vi "TSI Bench Single Socket CPV Sweeps Ver1.0.vi"() -> ()   [LabVIEW 2017]
uses:
  <vilib>/Utility/file.llb/Read Delimited Spreadsheet (DBL).vi
  <instrlib>/Agilent E364X Series/Agilent E364X Series.lvlib
  <instrlib>/Agilent E4980/Agilent E4980.lvlib
  <instrlib>/Keithley 2000/Keithley 2000.lvlib
panel:
  out "Cycles":string="2000"
  in  "Tab Control":enum32{"Control"}(tab)
  in  "T- CAP(fF)":dbl[](array[numeric])=[100.0, 2968.75]
  out "Diff DCAP":dbl[](array[numeric])=[0.0, 158.76451612903202, 128.65967741935475, 83.51039999999999, 79.098, 80.17639999999999, 81.14560000000002, 79.77199999999999, 91.06439999999998, 80.7144, 80.3784, 79.76879999999998, 80.59799999999998, 91.3732, 90.2772]
  out "IDD ON (uA)":string
  out "I_Stdby (uA)":string
  out "CMax(fF)":dbl
  in  "Cycle?":bool=TRUE
  out "Cycles  No":i32=2000
  out "CMin (fF)":dbl=255.30700000000002
  in  "TP":string="TSI Bench Single Socket CPV Sweep Ver1.0"
  out "Error Out":errorcluster={"status"=FALSE, "code"=1073676407, "source"="VISA Open in Agilent E364X Series.lvlib:Initialize.vi->WS1021 Screen Parts Bench Test Ver1.4.vi"}
  in  "Base Path":path=path "C:/TSI Material"
  out "Status":string="Save Data..."
  in  "Tab Control 2":T1(tab)=enum."Input Info"
  in  "AGE364X":refnum<visa-resource-name>="GPIB0::6::INSTR"
  in  "VDD/VIO":dbl[](array[numeric])=[3.3, 1.8]
  in  "I_Limit (mA)":dbl=20.0 format="%.2p"
  in  "Select CPV":i32(ring)=17 items=["CP 24V", "CP 26V", "CP 28V", "CP 30V", "CP 31V", "CP 32V", "CP 33V", "CP 34V", "CP 35V", "CP 36V", "CP 37V", "CP 38V", "CP 39V", "CP 40V", "CP 41V", "CP 42V", "CP 43V", "CP 44V", "CP 45V", "CP 46V", "CP 47V", "CP 48V", "CP 49V", "CP 50V", "CP 51V", "CP 52V", "CP 53V", "CP 54V", "CP 56V", "CP 58V", "CP 60V", "CP 62V"]
  in  "Settings":bool
  in  "Comport Setting":refnum<visa-resource-name>="COM8"
  in  "Manual Write":string
  in  "Send":bool
  in  "No of Cycles":i32=2000
  in  "Type (0: Cp-D)":u16(ring)=1 items=["Cp-D", "Cp-Q", "Cp-G", "Cp-Rp", "Cs-D", "Cs-Q", "Cs-Rs", "Lp-D", "Lp-Q", "Lp-G", "Lp-Rp", "Ls-D", "Ls-Q", "Ls-Rs", "R-X", "Z-thd", "Z-thr", "G-B", "Y-thd", "Y-thr"]
  in  "Auto Range":bool=TRUE
  in  "AG4980A":refnum<visa-resource-name>="GPIB0::17::INSTR"
  in  "KE2000":refnum<visa-resource-name>="GPIB0::9::INSTR"
  in  "Process Stop Button":bool
  in  "Read X, Y Setting":string[](array[string])=["68", "69"]
  in  "Stop":bool
  in  "Error In":errorcluster
  in  "CP CYC":bool
  in  "VDD":bool
  in  "Capacitance":bool
  in  "Info":T2={"Lot"="3127C", "Wafer"="11", "Package"="BC_C", "Device"="1"}
  out "IDD":cluster{dbl[], dbl[]}(graph)
  out "Cap Plot":cluster{dbl[], dbl[]}(graph)
  # "WiSpry Inc 20 Fairbanks \nSte 198 Irvine CA 92618\n\n\n\n\nRev Date = 11/11/2020\nTP:  TSI Bench Single Socket CPV Sweep Ver1.0\nLabVIEW 2017"
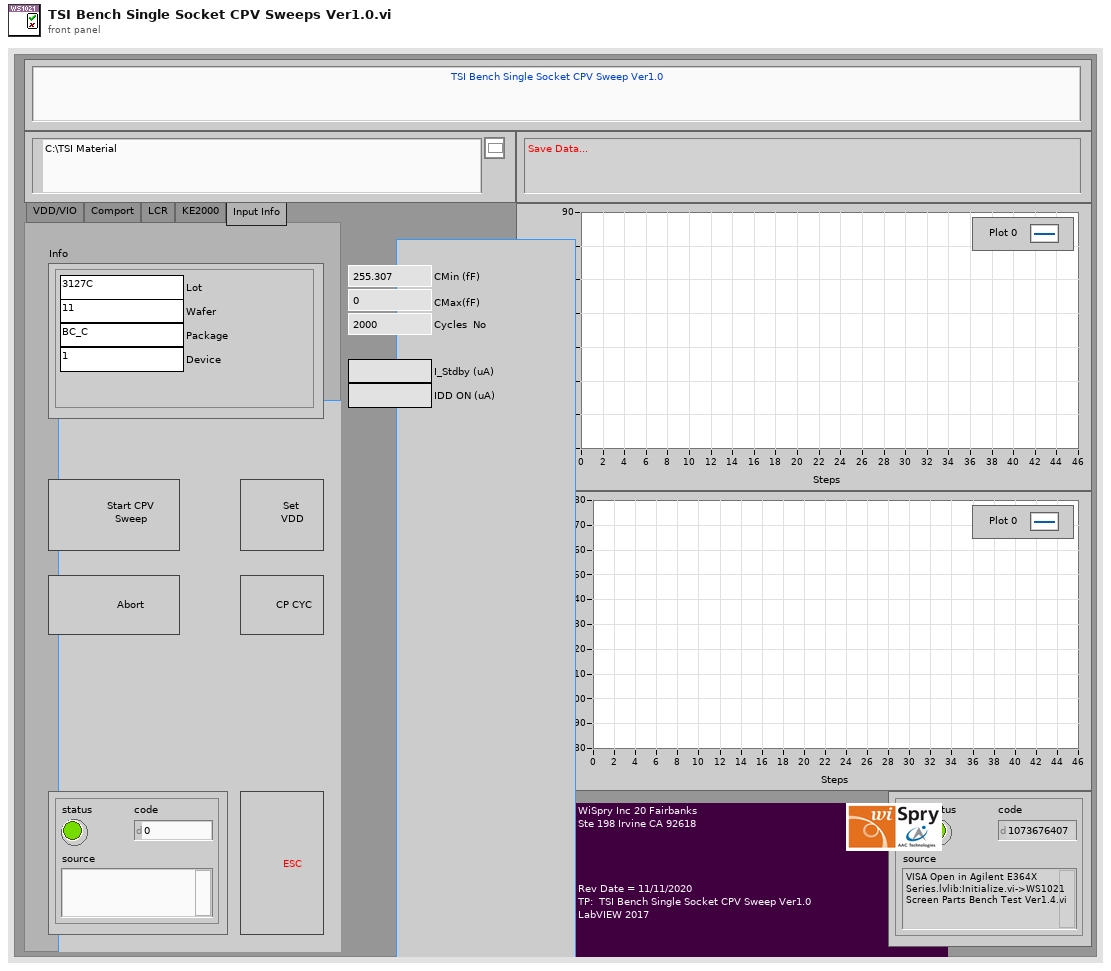
[diagram p1: front panel]
types:
  T1 = enum32{"VDD/VIO", "Comport", "LCR", "KE2000", "Input Info"}
  T2 = cluster{"Lot":string, "Wafer":string, "Package":string, "Device":string}
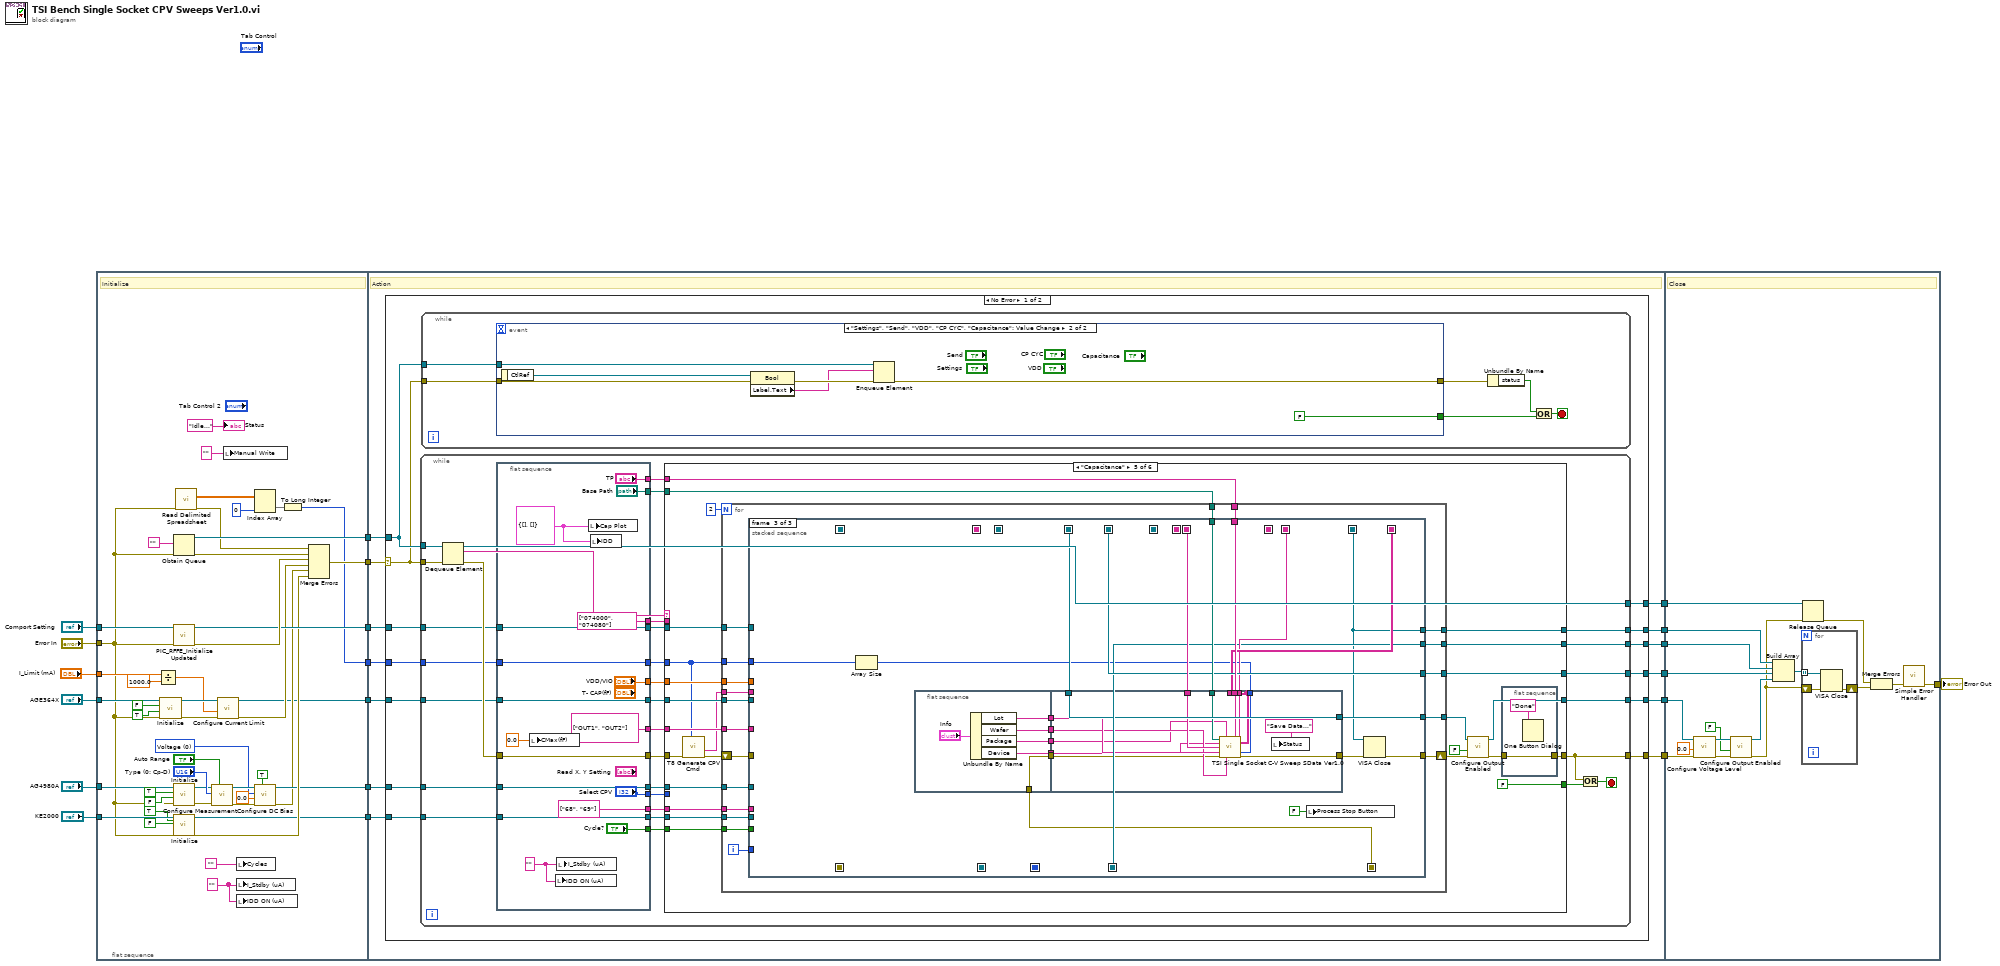
[diagram p0: block diagram]
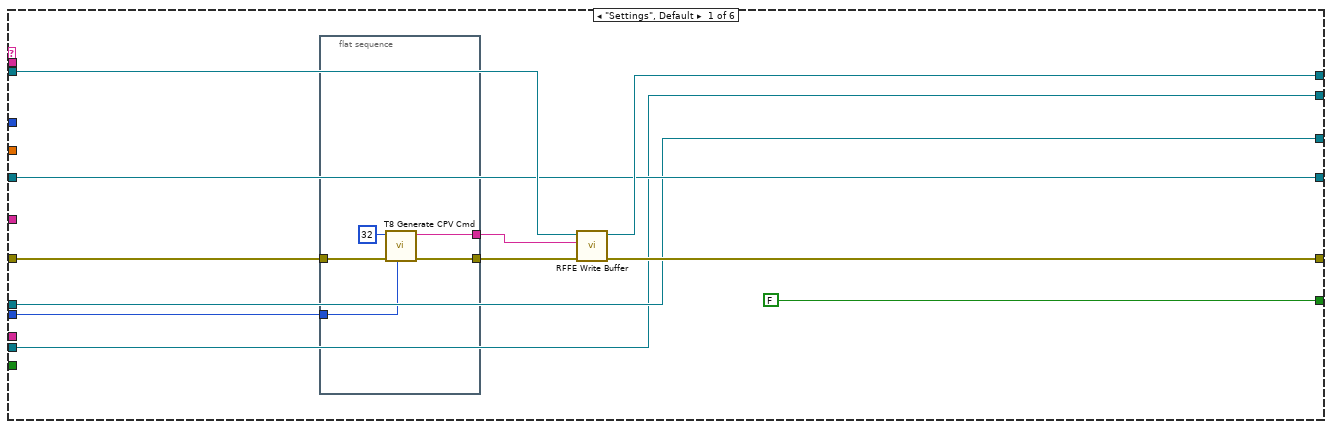
[diagram p2: hidden frame]
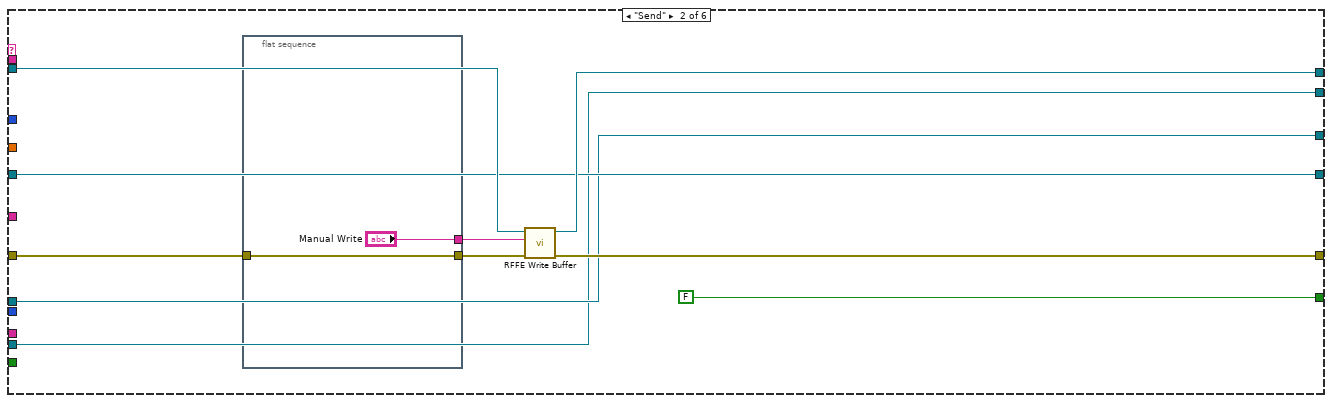
[diagram p3: hidden frame]
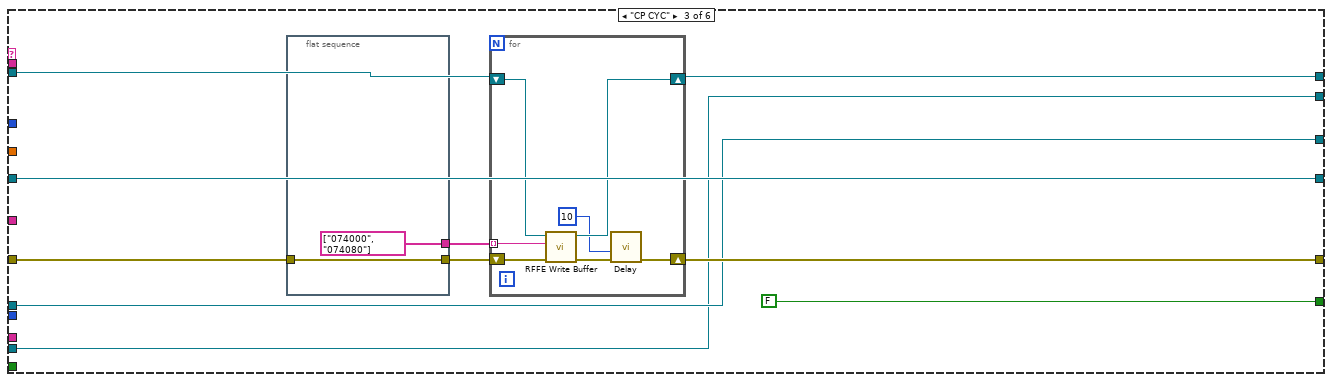
[diagram p4: hidden frame]
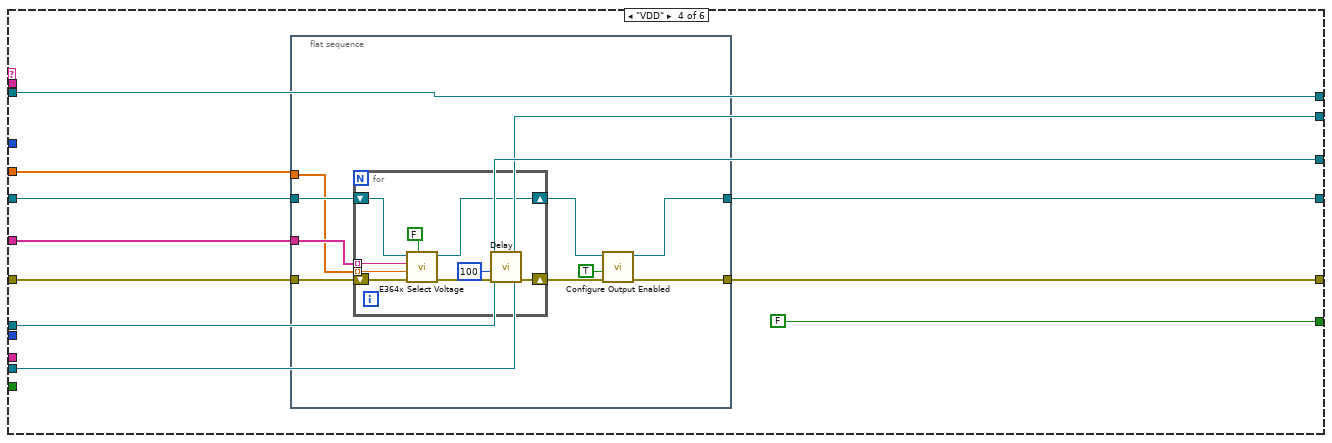
[diagram p5: hidden frame]
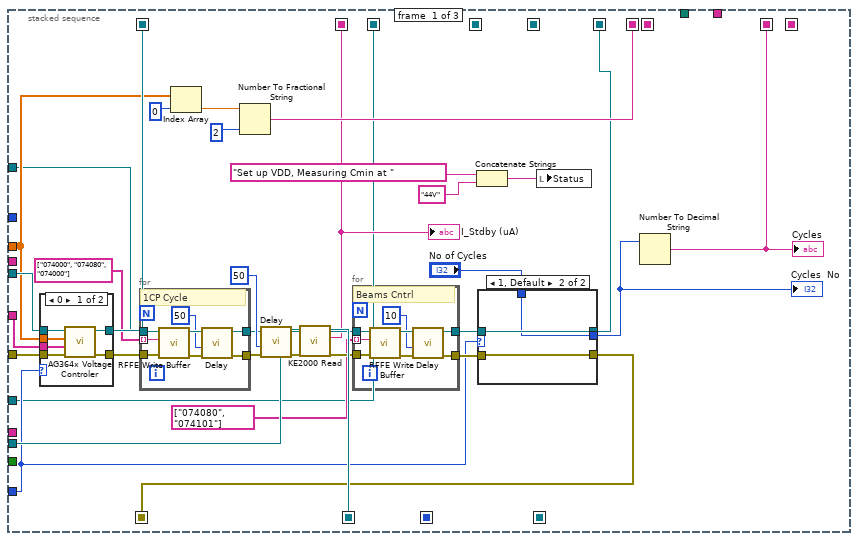
[diagram p6: hidden frame]
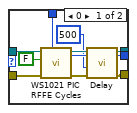
[diagram p8: hidden frame]
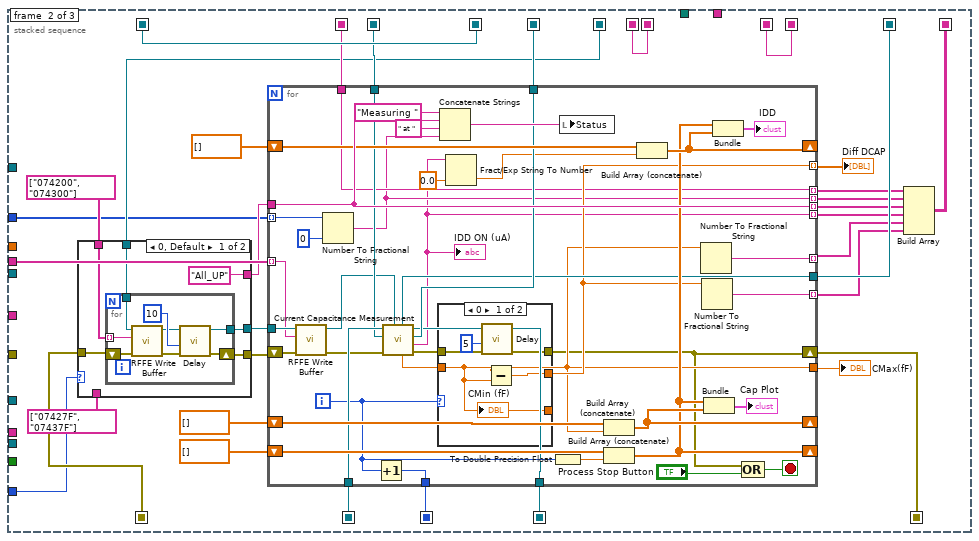
[diagram p9: hidden frame]
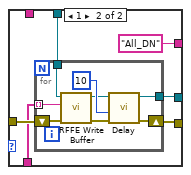
[diagram p10: hidden frame]
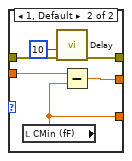
[diagram p11: hidden frame]
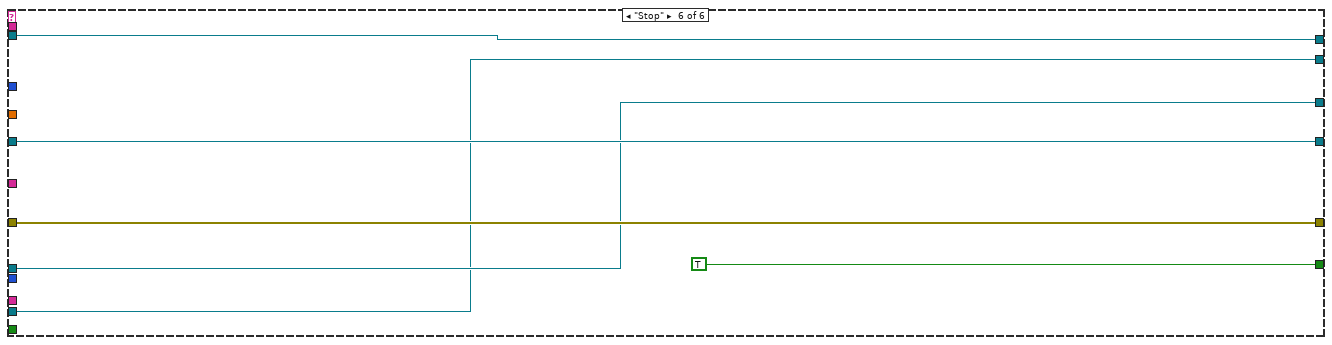
[diagram p12: hidden frame]
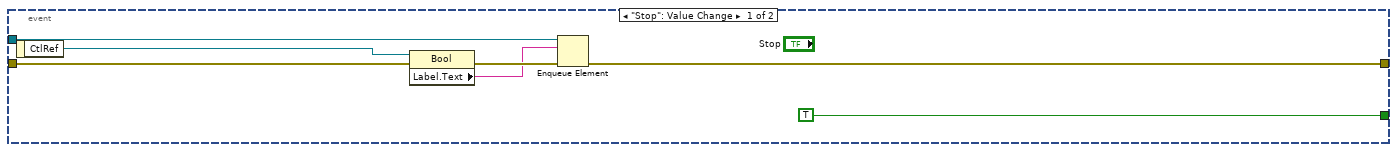
[diagram p13: hidden frame]
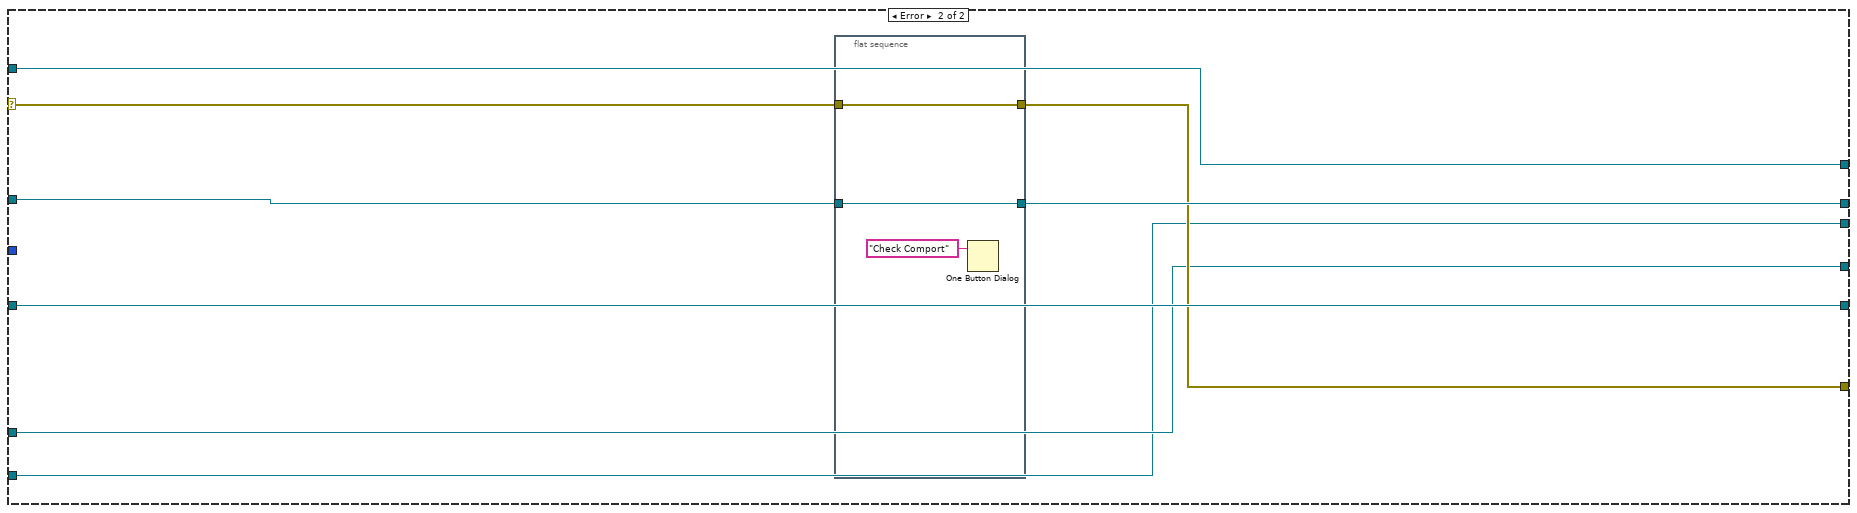
[diagram p14: hidden frame]
diagram:
  n1 = flat-sequence {
    tunnel: "Error In" -> [w23]
    tunnel: [w63] -> w19
    tunnel: [w65] -> w18
    tunnel: "Comport Setting" -> [w64]
    tunnel: [w60] -> w15
    tunnel: "AGE364X" -> [w58]
    tunnel: [w31] -> w11
    tunnel: "AG4980A" -> [w49]
    tunnel: [w41] -> w7
    tunnel: "KE2000" -> [w45]
    tunnel: [w42] -> w4
    tunnel: "I_Limit (mA)" -> [w30]
    tunnel: [w21] -> w1
    tunnel: w19 -> [w75]
    tunnel: w18 -> [w79]
    tunnel: [w78] -> w17
    tunnel: w15 -> [w77]
    tunnel: [w76] -> w14
    tunnel: w11 -> [w74]
    tunnel: [w73] -> w10
    tunnel: [w72] -> w9
    tunnel: w7 -> [w71]
    tunnel: [w70] -> w6
    tunnel: w4 -> [w69]
    tunnel: [w68] -> w3
    tunnel: w1 -> [w67]
    tunnel: w17 -> [w533]
    tunnel: w14 -> [w519]
    tunnel: [w532] -> w13
    tunnel: w10 -> [w528]
    tunnel: w9 -> [w524]
    tunnel: w6 -> [w521]
    tunnel: w3 -> [w518]
    frame #0 {
      w27 = "" ("I_Stdby (uA)")
      w38 = u16 0 items=["Voltage", "Current"] ("DC Bias Type (0: Voltage)")
      # "Initialize"
      n2 = Divide(x=w30, y=1000.0) -> (x/y=w28:dbl)
      n3 = call <instrlib>:"Initialize.vi"("error in (no error)"=w23, "ID Query (T: Query)"=TRUE, "Reset Device (T: Reset)"=FALSE, "VISA resource name"=w58) -> ("error out"=w33:errorcluster, "VISA resource name out"=w34:refnum<visa-resource-name>)  [unwired: 6 in]
      n4 = Obtain Queue(element data type="", error in (no error)=w23) -> (queue out=w65:refnum<queue>, error out=w62:errorcluster)  [unwired: 3 in, 1 out]
      n5 = call "PIC_RFFE_Initialize Updated.vi"("error in"=w23, "VISA In"=w64) -> ("error out"=w61:errorcluster, "VISA Out"=w60:refnum<visa-resource-name>)  [unwired: 8 in]
      n6 = call <instrlib>:"Initialize.vi"("error in (no error)"=w23, "Reset (True)"=FALSE, "ID Query (True)"=TRUE, "VISA resource name"=w49) -> ("error out"=w53:errorcluster, "VISA resource name out"=w52:refnum<visa-resource-name>)  [unwired: 6 in]
      n7 = call <instrlib>:"Initialize.vi"("VISA resource name"=w45, "ID Query? (T: Check)"=TRUE, "Reset? (T: Reset)"=FALSE, "error in (no error)"=w23) -> ("VISA resource name out"=w42:refnum<visa-resource-name>, "error out"=w46:errorcluster)  [unwired: 14 in]
      n8 = call-poly <vilib>:"Read Delimited Spreadsheet.vi"("error in (no error)"=w23) -> ("all rows"=w26:dbl[][], "error out"=w22:errorcluster)  [unwired: 9 in, 4 out]
      n9 = call <instrlib>:"Configure Measurement.vi"("Enable Auto Range (T:Enable)"="Auto Range", "error in (no error)"=w53, "Function (0: Cp-D)"="Type (0: Cp-D)", "VISA resource name"=w52) -> ("error out"=w37:errorcluster, "VISA resource name out"=w40:refnum<visa-resource-name>)  [unwired: 6 in]
      n10 = call <instrlib>:"Configure Current Limit.vi"("error in (no error)"=w33, "Current Limit (0.0 Amps)"=w28, "VISA resource name"=w34) -> ("error out"=w32:errorcluster, "VISA resource name out"=w31:refnum<visa-resource-name>)  [unwired: 7 in]
      n11 = local write "Manual Write"("" ("Manual Write")) -> ()
      n12 = local write "Cycles"("") -> ()
      n13 = local write "I_Stdby (uA)"(w27) -> ()
      n14 = local write "IDD ON (uA)"(w27) -> ()
      n15 = Index Array(array=w26, index (col)=0 ("disabled index (col)")) -> (element=w24:dbl[])  [unwired: 1 in]
      n16 = call <instrlib>:"Configure DC Bias.vi"("DC Bias State (F:Disable)"=TRUE, "error in (no error)"=w37, "DC Bias Level (0.0 V)"=0.0, "DC Bias Type (0: Voltage)"=w38, "VISA resource name"=w40) -> ("error out"=w36:errorcluster, "VISA resource name out"=w41:refnum<visa-resource-name>)  [unwired: 5 in]
      n17 = To Long Integer(number=w24) -> (32bit integer=w21:i32[])
      n18 = Merge Errors(w22, w62, w61, w32, w36, w46) -> (w63:errorcluster)
      "Status" <- "Idle..." ("Status")
    }
    frame #1 {
      # "Action"
      n19 = case shown="No Error" w75 {
        selector: w75 -> [w88 w509]
        tunnel: w79 -> [w92 w511]
        tunnel: [w91 w511] -> w78
        tunnel: w77 -> [w90 w513]
        tunnel: [w89 w512] -> w76
        tunnel: w74 -> [w87 w510]
        tunnel: [w86 w508] -> w73
        tunnel: [w85 w510] -> w72
        tunnel: w71 -> [w84 w507]
        tunnel: [w83 w507] -> w70
        tunnel: w69 -> [w82 w506]
        tunnel: [w81 w506] -> w68
        tunnel: w67 -> [w80 _]
        frame No Error {
          n20 = while {
            tunnel: w92 -> [w123]
            tunnel: w88 -> [w122]
            tunnel: [w116] -> w91
            tunnel: w90 -> [w115]
            tunnel: [w113] -> w89
            tunnel: w87 -> [w112]
            tunnel: [w109] -> w85
            tunnel: [w104] -> w86
            tunnel: w84 -> [w107]
            tunnel: [w105] -> w83
            tunnel: w82 -> [w100]
            tunnel: [w98] -> w81
            tunnel: w80 -> [w94]
            stop <- w118 stop-if-true
            n21 = Dequeue Element(queue=w123, error in (no error)=w122) -> (queue out=w116:refnum<queue>, element=w121:string, error out=w120:errorcluster)  [unwired: 1 in, 1 out]
            n22 = flat-sequence {
              tunnel: w120 -> [w485]
              tunnel: [w485] -> w119
              tunnel: w115 -> [w484]
              tunnel: [w484] -> w114
              tunnel: w112 -> [w483]
              tunnel: [w483] -> w111
              tunnel: [string[] ["OUT1", "OUT2"]] -> w110
              tunnel: ["VDD/VIO"] -> w108
              tunnel: w107 -> [w481]
              tunnel: [w481] -> w106
              tunnel: ["Base Path"] -> w103
              tunnel: ["TP"] -> w102
              tunnel: ["Select CPV"] -> w101
              tunnel: w100 -> [w477]
              tunnel: [w477] -> w99
              tunnel: [string[] ["074000", "074080"]] -> w97
              tunnel: ["Cycle?"] -> w96
              tunnel: [string[] ["68", "69"]] -> w95
              tunnel: [w470] -> w93
              tunnel: w94 -> [w470]
              frame #0 {
                w472 = "" ("I_Stdby (uA)")
                w473 = cluster{dbl[], dbl[]} {[], []} ("Cap Plot")
                n23 = local write "CMax(fF)"(0.0 ("CMax(fF)")) -> ()
                n24 = local write "IDD ON (uA)"(w472) -> ()
                n25 = local write "I_Stdby (uA)"(w472) -> ()
                n26 = local write "Cap Plot"(w473) -> ()
                n27 = local write "IDD"(w473) -> ()
              }
            }
            n28 = case shown="\"Capacitance\"" w121 {
              tunnel: w119 -> [w134 w146 w158 w178 w203 w468]
              tunnel: [w131 w149 w161 w177 w206 w468] -> w104
              tunnel: [FALSE FALSE FALSE FALSE FALSE TRUE] -> w117
              tunnel: w114 -> [w130 w147 w159 w179 w217 w466]
              tunnel: [w129 w148 w160 w179 w216 w466] -> w113
              tunnel: w111 -> [w127 w142 w154 w176 w211 w465]
              tunnel: w110 -> [_ _ _ w175 w222 _]
              tunnel: [w127 w142 w154 w174 w205 w465] -> w109
              tunnel: w108 -> [_ _ _ w173 w223 _]
              tunnel: w106 -> [w126 w141 w153 w172 w213 w464]
              tunnel: [w126 w141 w153 w172 w212 w464] -> w105
              tunnel: w103 -> [_ _ _ _ w220 _]
              tunnel: w102 -> [_ _ _ _ w219 _]
              tunnel: w101 -> [w125 _ _ _ _ _]
              tunnel: w99 -> [w124 w140 w152 w171 w215 w463]
              tunnel: [w124 w140 w152 w171 w214 w463] -> w98
              tunnel: w97 -> [_ _ _ _ _ _]
              tunnel: w96 -> [_ _ _ _ w218 _]
              tunnel: w95 -> [_ _ _ _ w204 _]
              tunnel: w93 -> [_ _ _ _ w199 _]
              frame "Settings", Default {
                n29 = flat-sequence {
                  tunnel: w134 -> [w139]
                  tunnel: [w138] -> w132
                  tunnel: [w137] -> w128
                  tunnel: w125 -> [w135]
                  frame #0 {
                    n30 = call "T8 Generate CPV Cmd.vi"("Select CPV"=w135, "Error In"=w139, "Steps"=32) -> ("Error Out"=w138:errorcluster, "Cmd Send out"=w137:string)  [unwired: 5 in, 2 out]
                  }
                }
                n31 = call "RFFE Write Buffer.vi"("error in (no error)"=w132, "write buffer"=w128, "VISA resource name"=w130) -> ("error out"=w131:errorcluster, "VISA resource name out"=w129:refnum<visa-resource-name>)  [unwired: 7 in]
              }
              frame "Send" {
                n32 = flat-sequence {
                  tunnel: w146 -> [w151]
                  tunnel: [w151] -> w145
                  tunnel: ["Manual Write"] -> w144
                  frame #0 {
                  }
                }
                n33 = call "RFFE Write Buffer.vi"("error in (no error)"=w145, "write buffer"=w144, "VISA resource name"=w147) -> ("error out"=w149:errorcluster, "VISA resource name out"=w148:refnum<visa-resource-name>)  [unwired: 7 in]
              }
              frame "CP CYC" {
                n34 = flat-sequence {
                  tunnel: w158 -> [w170]
                  tunnel: [w170] -> w157
                  tunnel: [string[] ["074000", "074080"]] -> w156
                  frame #0 {
                  }
                }
                n35 = for {
                  tunnel: w156 -> [w165] mode=indexing
                  shift-right: [w168] -> w160
                  shift-left: w159 -> [w167]
                  shift-right: [w164] -> w161
                  shift-left: w157 -> [w166]
                  n36 = call "RFFE Write Buffer.vi"("error in (no error)"=w166, "write buffer"=w165, "VISA resource name"=w167) -> ("error out"=w163:errorcluster, "VISA resource name out"=w168:refnum<visa-resource-name>)  [unwired: 7 in]
                  n37 = call "Delay.vi"("error in (no error)"=w163, "Delay"=u32 10) -> ("error out"=w164:errorcluster)  [unwired: 9 in]
                }
              }
              frame "VDD" {
                n38 = flat-sequence {
                  tunnel: [w183] -> w174
                  tunnel: [w184] -> w177
                  tunnel: w176 -> [w188]
                  tunnel: w178 -> [w189]
                  tunnel: w175 -> [w187]
                  tunnel: w173 -> [w186]
                  frame #0 {
                    n39 = for {
                      shift-right: [w197] -> w185
                      shift-left: w189 -> [w198]
                      shift-right: [w190] -> w181
                      shift-left: w188 -> [w194]
                      tunnel: w187 -> [w193] mode=indexing
                      tunnel: w186 -> [w192] mode=indexing
                      n40 = call "E364x Select Voltage.vi"("Output Enabled (F: Off)"=FALSE, "error in"=w198, "Level (0.0 Volts)"=w192, "Output"=w193, "VISA in"=w194) -> ("error out"=w196:errorcluster, "VISA Out"=w190:refnum<visa-resource-name>)  [unwired: 5 in]
                      n41 = call "Delay.vi"("error in (no error)"=w196, "Delay"=u32 100) -> ("error out"=w197:errorcluster)  [unwired: 9 in]
                    }
                    n42 = call <instrlib>:"Configure Output Enabled.vi"("error in (no error)"=w185, "Output Enabled (F: Off)"=TRUE, "VISA resource name"=w181) -> ("error out"=w184:errorcluster, "VISA resource name out"=w183:refnum<visa-resource-name>)  [unwired: 7 in]
                  }
                }
              }
              frame "Capacitance" {
                n43 = call "T8 Generate CPV Cmd.vi"("CP For Test"=w199, "Error In"=w203) -> ("Error Out"=w202:errorcluster, "Cmd Select"=w201:string[])  [unwired: 6 in, 2 out]
                n44 = for {
                  N: 2 -> [_]
                  tunnel: w223 -> [w244]
                  tunnel: w222 -> [w243]
                  tunnel: w220 -> [w241]
                  tunnel: w219 -> [w239]
                  tunnel: w218 -> [w238]
                  shift-right: [w240] -> w209
                  shift-left: w202 -> [w242]
                  tunnel: w217 -> [w237]
                  tunnel: [w236] -> w216
                  tunnel: w215 -> [w235]
                  tunnel: [w234] -> w214
                  tunnel: w213 -> [w233]
                  tunnel: [w232] -> w212
                  tunnel: w211 -> [w231]
                  tunnel: [w230] -> w208
                  tunnel: w204 -> [w228]
                  tunnel: w201 -> [w227]
                  tunnel: w199 -> [w226]
                  i -> [w229]
                  n45 = stacked-sequence {
                    seq-local: [w246 _ _] -> [_ w323 _]
                    seq-local: [w274 _ _] -> [_ w342 _]
                    seq-local: [_ w344 _] -> [_ _ w433]
                    seq-local: [_ w343 _] -> [_ _ w426]
                    seq-local: [_ w342 _] -> [_ _ w442]
                    seq-local: [w269 _ _] -> [_ w341 _]
                    seq-local: [_ w341 _] -> [_ _ w438]
                    seq-local: [w248 _ _] -> [_ w340 _]
                    seq-local: [_ w339 _] -> [_ _ w437]
                    seq-local: [w245 _ _] -> [_ w322 _]
                    seq-local: [_ w337 _] -> [_ _ w436]
                    seq-local: [w263 _ _] -> [_ w336 _]
                    seq-local: [_ w336 _] -> [_ _ w435]
                    seq-local: [w258 _ _] -> [_ w330 _]
                    seq-local: [_ w329 _] -> [_ _ w434]
                    seq-local: [w252 _ _] -> [_ w326 _]
                    seq-local: [_ w324 _] -> [_ _ _]
                    tunnel: w231 -> [w277 _ _]
                    tunnel: w244 -> [w270 _ _]
                    tunnel: w243 -> [w275 _ _]
                    tunnel: w242 -> [w276 _ _]
                    tunnel: w237 -> [w266 _ _]
                    tunnel: w233 -> [w248 _ _]
                    tunnel: [_ _ w441] -> w230
                    tunnel: w241 -> [_ _ w440]
                    tunnel: [_ _ w431] -> w240
                    tunnel: w239 -> [_ _ w439]
                    tunnel: [_ _ w437] -> w232
                    tunnel: [_ _ w433] -> w236
                    tunnel: w235 -> [w259 _ _]
                    tunnel: [_ _ w434] -> w234
                    tunnel: w238 -> [_ _ _]
                    tunnel: w229 -> [w249 w319 _]
                    tunnel: w228 -> [_ _ _]
                    tunnel: w227 -> [_ w320 _]
                    tunnel: w226 -> [_ w313 w423]
                    frame #0 {
                      n46 = case shown="0" w249 {
                        tunnel: w277 -> [w283 w284]
                        tunnel: w276 -> [w282 w285]
                        tunnel: w275 -> [w281 _]
                        tunnel: [w280 w284] -> w274
                        tunnel: w270 -> [w279 _]
                        tunnel: [w278 w285] -> w267
                        frame 0 {
                          n47 = call "AG364x Voltage Controler.vi"("error in (no error)"=w282, "Select CH"=w281, "VDD/VIO"=w279, "VISA In"=w283) -> ("error out"=w278:errorcluster, "VISA Out"=w280:refnum<visa-resource-name>)  [unwired: 6 in]
                        }
                        frame 1, Default {
                        }
                      }
                      n48 = for {
                        tunnel: [w307] -> w261
                        tunnel: string[] ["074000", "074080", "074000"] -> [w311] mode=indexing
                        tunnel: w267 -> [w310]
                        tunnel: w266 -> [w309]
                        tunnel: [w308] -> w254
                        # "1CP Cycle"
                        n49 = call "RFFE Write Buffer.vi"("error in (no error)"=w310, "write buffer"=w311, "VISA resource name"=w309) -> ("error out"=w306:errorcluster, "VISA resource name out"=w308:refnum<visa-resource-name>)  [unwired: 7 in]
                        n50 = call "Delay.vi"("error in (no error)"=w306, "Delay"=u32 50) -> ("error out"=w307:errorcluster)  [unwired: 9 in]
                      }
                      n51 = Index Array(array=w270, index=0) -> (element=w273:dbl)
                      n52 = Number To Fractional String(number=w273, precision (6)=i16 2) -> (F-format string=w269:string)  [unwired: 2 in]
                      n53 = call "Delay.vi"("error in (no error)"=w261, "Delay"=u32 50) -> ("error out"=w262:errorcluster)  [unwired: 9 in]
                      n54 = call "KE2000 Read.vi"("error in (no error)"=w262, "VISA resource name"=w259) -> ("error out"=w256:errorcluster, "uA"=w252:string, "VISA resource name out"=w258:refnum<visa-resource-name>)  [unwired: 7 in]
                      "I_Stdby (uA)" <- w252
                      n55 = for {
                        tunnel: [w288] -> w257
                        tunnel: string[] ["074080", "074101"] -> [w292] mode=indexing
                        tunnel: w256 -> [w291]
                        tunnel: w254 -> [w290]
                        tunnel: [w289] -> w253
                        # "Beams Cntrl"
                        n56 = call "RFFE Write Buffer.vi"("error in (no error)"=w291, "write buffer"=w292, "VISA resource name"=w290) -> ("error out"=w287:errorcluster, "VISA resource name out"=w289:refnum<visa-resource-name>)  [unwired: 7 in]
                        n57 = call "Delay.vi"("error in (no error)"=w287, "Delay"=u32 10) -> ("error out"=w288:errorcluster)  [unwired: 9 in]
                      }
                      n58 = Concatenate Strings("Set up VDD, Measuring Cmin at " ("Status"), "44V" ("string")) -> (w250:string)
                      n59 = case shown="1, Default" w249 {
                        tunnel: w253 -> [w300 w304]
                        tunnel: w257 -> [w299 w302]
                        tunnel: [w294 w302] -> w246
                        tunnel: [w298 w304] -> w245
                        tunnel: [w297 w303] -> w264
                        tunnel: "No of Cycles" -> [w296 w303]
                        frame 0 {
                          n60 = call "WS1021 PIC RFFE Cycles.vi"("No of Cycles"=w296, "Error In"=w299, "Init"=FALSE, "VISA In"=w300) -> ("Error Out"=w295:errorcluster, "VISA Out"=w298:refnum<visa-resource-name>, "Cycles Completed"=w297:i32)  [unwired: 5 in]
                          n61 = call "Delay.vi"("error in (no error)"=w295, "Delay"=u32 500) -> ("error out"=w294:errorcluster)  [unwired: 9 in]
                        }
                        frame 1, Default {
                        }
                      }
                      "Cycles  No" <- w264
                      n62 = local write "Status"(w250) -> ()
                      n63 = Number To Decimal String(number=w264) -> (decimal integer string=w263:string)  [unwired: 1 in]
                      "Cycles" <- w263
                    }
                    frame #1 {
                      n64 = case shown="0, Default" w319 {
                        tunnel: w323 -> [w350 w363]
                        tunnel: w322 -> [w346 w362]
                        tunnel: [w348 w361] -> w321
                        tunnel: [w349 w360] -> w318
                        tunnel: string[] ["074200", "074300"] -> [w347 _]
                        tunnel: string[] ["07427F", "07437F"] -> [_ w359]
                        tunnel: ["All_UP" "All_DN"] -> w315
                        frame 0, Default {
                          n65 = for {
                            shift-right: [w355] -> w349
                            shift-left: w350 -> [w357]
                            tunnel: w346 -> [w353]
                            tunnel: [w352] -> w348
                            tunnel: w347 -> [w351] mode=indexing
                            n66 = call "RFFE Write Buffer.vi"("error in (no error)"=w357, "write buffer"=w351, "VISA resource name"=w353) -> ("error out"=w356:errorcluster, "VISA resource name out"=w352:refnum<visa-resource-name>)  [unwired: 7 in]
                            n67 = call "Delay.vi"("error in (no error)"=w356, "Delay"=u32 10) -> ("error out"=w355:errorcluster)  [unwired: 9 in]
                          }
                        }
                        frame 1 {
                          n68 = for {
                            shift-right: [w368] -> w360
                            shift-left: w363 -> [w370]
                            tunnel: w362 -> [w366]
                            tunnel: [w365] -> w361
                            tunnel: w359 -> [w364] mode=indexing
                            n69 = call "RFFE Write Buffer.vi"("error in (no error)"=w370, "write buffer"=w364, "VISA resource name"=w366) -> ("error out"=w369:errorcluster, "VISA resource name out"=w365:refnum<visa-resource-name>)  [unwired: 7 in]
                            n70 = call "Delay.vi"("error in (no error)"=w369, "Delay"=u32 10) -> ("error out"=w368:errorcluster)  [unwired: 9 in]
                          }
                        }
                      }
                      n71 = for {
                        shift-right: [w371] -> w343
                        shift-left: w318 -> [w388]
                        tunnel: [w382] -> w344
                        tunnel: [w383] -> w339
                        tunnel: w340 -> [w396]
                        tunnel: w315 -> [w409]
                        tunnel: [w405] -> w338 mode=indexing
                        tunnel: [w409] -> w327 mode=indexing
                        tunnel: [w376] -> w335 mode=indexing
                        tunnel: [w380] -> w334 mode=indexing
                        tunnel: [w374] -> w328 mode=indexing
                        shift-right: [w400] -> _
                        shift-left: dbl[] [] -> [w407]
                        shift-right: [w402] -> _
                        shift-left: dbl[] [] -> [w406]
                        shift-right: [w399] -> _
                        shift-left: dbl[] [] -> [w404]
                        tunnel: w330 -> [w397]
                        tunnel: [w381] -> w329
                        tunnel: [w394] -> w314 mode=indexing
                        tunnel: w326 -> [w379]
                        tunnel: [w379] -> w325 mode=indexing
                        tunnel: [w375] -> w312
                        tunnel: [w389] -> w324
                        tunnel: w321 -> [w385]
                        tunnel: w320 -> [w384] mode=indexing
                        tunnel: w313 -> [w377] mode=indexing
                        i -> [w390]
                        stop <- w391 stop-if-true
                        n72 = call "RFFE Write Buffer.vi"("error in (no error)"=w388, "write buffer"=w384, "VISA resource name"=w385) -> ("error out"=w387:errorcluster, "VISA resource name out"=w386:refnum<visa-resource-name>)  [unwired: 7 in]
                        n73 = Number To Fractional String(number=w377, precision (6)=i16 0) -> (F-format string=w376:string)  [unwired: 2 in]
                        n74 = Increment(x=w390) -> (x+1=w389:i32)
                        n75 = call "Current Capacitance Measurement.vi"("RFFE In"=w386, "Error In"=w387, "E4980A LCR In"=w396, "KE2000 In"=w397) -> ("Error Out"=w395:errorcluster, "uA"=w374:string, "E4980A LCR Out"=w383:refnum<visa-resource-name>, "KE2000 Out"=w381:refnum<visa-resource-name>, "Cap(fF)"=w375:dbl, "RFFE Out"=w382:refnum<visa-resource-name>)  [unwired: 2 in]
                        "IDD ON (uA)" <- w374
                        n76 = case shown="0" w390 {
                          tunnel: [w415 w421] -> w371
                          tunnel: w395 -> [w414 w420]
                          tunnel: w375 -> [w412 w416]
                          tunnel: [w412 w417] -> _
                          tunnel: [w411 w418] -> w380
                          frame 0 {
                            n77 = call "Delay.vi"("error in (no error)"=w414, "Delay"=u32 5) -> ("error out"=w415:errorcluster)  [unwired: 9 in]
                            n78 = Subtract(x=w412, y=w412) -> (x-y=w411:dbl)
                            "CMin (fF)" <- w412
                          }
                          frame 1, Default {
                            n79 = local read "CMin (fF)"() -> (w417:dbl)
                            n80 = call "Delay.vi"("error in (no error)"=w420, "Delay"=u32 10) -> ("error out"=w421:errorcluster)  [unwired: 9 in]
                            n81 = Subtract(x=w416, y=w417) -> (x-y=w418:dbl)
                          }
                        }
                        n82 = Concatenate Strings("Measuring " ("Status"), w409, " at " ("string"), w376) -> (w408:string)
                        n83 = Fract/Exp String To Number(string=w374, default (0 dbl)=0.0 ("default (0 DBL)")) -> (number=w373:dbl)  [unwired: 2 in, 1 out]
                        n84 = To Double Precision Float(number=w390) -> (double precision float=w403:dbl)
                        n85 = local write "Status"(w408) -> ()
                        n86 = Build Array (concatenate)(w406, w375) -> (w402:dbl[])
                        n87 = Build Array (concatenate)(w404, w403) -> (w399:dbl[])
                        n88 = Build Array (concatenate)(w407, w373) -> (w400:dbl[])
                        n89 = Number To Fractional String(number=w375) -> (F-format string=w405:string)  [unwired: 3 in]
                        n90 = Number To Fractional String(number=w380) -> (F-format string=w394:string)  [unwired: 3 in]
                        n91 = Bundle(w399, w402) -> (→"Cap Plot":cluster{dbl[], dbl[]})  [unwired: 1 in]
                        n92 = Bundle(w399, w400) -> (→"IDD":cluster{dbl[], dbl[]})  [unwired: 1 in]
                        n93 = Compound Arithmetic op=OR(w371, "Process Stop Button") -> (w391:bool)
                      }
                      "Diff DCAP" <- w334
                      "CMax(fF)" <- w312
                      n94 = Build Array(w325, w335, w327, w328, w338, w314) -> (w337:string[][])
                    }
                    frame #2 {
                      n95 = Array Size(array=w423) -> (size(s)=w422:i32)
                      n96 = flat-sequence {
                        tunnel: [w447] -> w430
                        tunnel: [w446] -> w429
                        tunnel: [w445] -> w428
                        tunnel: [w444] -> w427
                        tunnel: w426 -> [w443]
                        tunnel: [w443] -> w425
                        tunnel: [w462] -> w441
                        tunnel: [w461] -> w432
                        tunnel: w442 -> [w462]
                        tunnel: w435 -> [w455]
                        tunnel: w436 -> [w457]
                        tunnel: [w457] -> _
                        tunnel: w438 -> [w458]
                        tunnel: w439 -> [w459]
                        tunnel: w440 -> [w460]
                        tunnel: w430 -> [w454]
                        tunnel: w429 -> [w453]
                        tunnel: w428 -> [w452]
                        tunnel: w427 -> [w451]
                        tunnel: w425 -> [w450]
                        tunnel: w422 -> [w449]
                        frame #0 {
                          n97 = Unbundle By Name("Info") -> ("Lot"=w447:string, "Wafer"=w446:string, "Package"=w444:string, "Device"=w445:string)
                        }
                        frame #1 {
                          n98 = call "TSI Single Socket C-V Sweep SData Ver1.0.vi"("Base Path"=w460, "Package"=w451, "Data In"=w457, "TP"=w459, "Cyc"=w455, "Cell"=w452, "VDD To PGR OTP"=w458, "Lot"=w454, "Index"=w449, "error in (no error)"=w450, "Wafer"=w453) -> ("error out"=w461:errorcluster)  [unwired: 4 in]
                          n99 = local write "Status"("Save Data..." ("Status")) -> ()
                        }
                      }
                      n100 = local write "Process Stop Button"(FALSE ("Process Stop Button")) -> ()
                      n101 = VISA Close(VISA resource name=w433, error in (no error)=w432) -> (error out=w431:errorcluster)
                    }
                  }
                }
                n102 = call <instrlib>:"Configure Output Enabled.vi"("error in (no error)"=w209, "Output Enabled (F: Off)"=FALSE, "VISA resource name"=w208) -> ("error out"=w207:errorcluster, "VISA resource name out"=w205:refnum<visa-resource-name>)  [unwired: 7 in]
                n103 = flat-sequence {
                  tunnel: w207 -> [w224]
                  tunnel: [w224] -> w206
                  frame #0 {
                    n104 = One Button Dialog(message="Done") -> ()  [unwired: 1 in, 1 out]
                  }
                }
              }
              frame "Stop" {
              }
            }
            n105 = Or(x=w104, y=w117) -> (x .or. y?=w118:bool)
          }
          n106 = while {
            tunnel: w88 -> [w491]
            tunnel: w92 -> [w490]
            stop <- w489 stop-if-true
            n107 = event shown="[1] \"Settings\", \"Send\", \"VDD\", \"CP CYC\", \"Capacitance\": Value Change" {
              selector: _ -> [_ _]
              dyn-events: _ -> [_ _]
              timeout: _ -> [_ _]
              tunnel: [TRUE ("Stop") FALSE ("Stop")] -> w487
              tunnel: w491 -> [w496 w503]
              tunnel: w490 -> [w498 w505]
              tunnel: [w493 w500] -> w486
              event "Stop": Value Change {
                n108 = event-data() -> ("CtlRef"=w497:refnum<vi>)  [unwired: 1 in]
                n109 = property class="Bool"(reference=w497, error in=w496) -> (error out=w495:errorcluster, "Label.Text"=w494:string)  [unwired: 1 out]
                n110 = Enqueue Element(queue=w498, element=w494, error in (no error)=w495) -> (error out=w493:errorcluster)  [unwired: 1 in, 2 out]
              }
              event "Settings", "Send", "VDD", "CP CYC", "Capacitance": Value Change {
                n111 = event-data() -> ("CtlRef"=w504:refnum<vi>)  [unwired: 1 in]
                n112 = property class="Bool"(reference=w504, error in=w503) -> (error out=w502:errorcluster, "Label.Text"=w501:string)  [unwired: 1 out]
                n113 = Enqueue Element(queue=w505, element=w501, error in (no error)=w502) -> (error out=w500:errorcluster)  [unwired: 1 in, 2 out]
              }
            }
            n114 = Unbundle By Name(w486) -> ("status"=w488:bool)
            n115 = Or(x=w488, y=w487) -> (x .or. y?=w489:bool)
          }
        }
        frame Error {
          n116 = flat-sequence {
            tunnel: [w515] -> w512
            tunnel: w513 -> [w515]
            tunnel: [w514] -> w508
            tunnel: w509 -> [w514]
            frame #0 {
              n117 = One Button Dialog(message="Check Comport") -> ()  [unwired: 1 in, 1 out]
            }
          }
        }
      }
    }
    frame #2 {
      # "Close"
      n118 = call <instrlib>:"Configure Voltage Level.vi"("error in (no error)"=w528, "Level (0.0 Volts)"=0.0, "VISA resource name"=w524) -> ("error out"=w527:errorcluster, "VISA resource name out"=w531:refnum<visa-resource-name>)  [unwired: 7 in]
      n119 = call <instrlib>:"Configure Output Enabled.vi"("error in (no error)"=w527, "Output Enabled (F: Off)"=FALSE, "VISA resource name"=w531) -> ("error out"=w517:errorcluster, "VISA resource name out"=w520:refnum<visa-resource-name>)  [unwired: 7 in]
      n120 = Build Array(w519, w518, w521, w520) -> (w522:refnum<visa-resource-name>[])
      n121 = for {
        tunnel: w522 -> [w536] mode=indexing
        shift-right: [w535] -> w523
        shift-left: w517 -> [w534]
        n122 = VISA Close(VISA resource name=w536, error in (no error)=w534) -> (error out=w535:errorcluster)
      }
      n123 = Release Queue(queue=w533, error in (no error)=w517) -> (error out=w526:errorcluster)  [unwired: 1 in, 2 out]
      n124 = Merge Errors(w526, w523) -> (w525:errorcluster)
      n125 = call <vilib>:"Simple Error Handler.vi"("error in (no error)"=w525) -> ("error out"=w532:errorcluster)  [unwired: 4 in, 4 out]
    }
  }
  "Error Out" <- w13
